vi "Write cRIO.vi"(10 "cRIO":T1={"Username"="admin", "IP Address"="140.252.33.38", "Path to ts_opensplice target"=path "/usr", "Path to ts_sal target"=path "/usr"}, 11 "FileTransfer in":refnum<class "FileTransfer.lvclass">) -> (3 "FileTransfer out":refnum<class "FileTransfer.lvclass">)   [LabVIEW 2016, in "FileTransfer.lvclass"]
uses:
  FileTransfer.lvclass
  Typedefs/cRIO.ctl
  FileTransfer.lvclass/FileTransfer.ctl
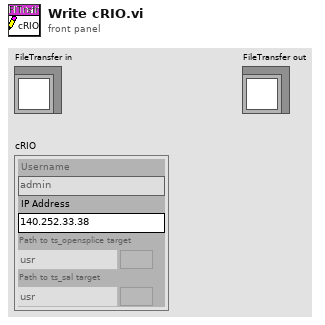
[diagram p1: front panel]
types:
  T1 = typedef "cRIO.ctl" = cluster{"Username":string, "IP Address":string, "Path to ts_opensplice target":path, "Path to ts_sal target":path}
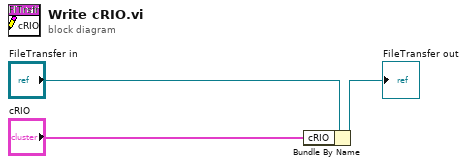
[diagram p0: block diagram]
diagram:
  n1 = Bundle By Name(cluster="FileTransfer in", "cRIO"="cRIO") -> (→"FileTransfer out":refnum<class "FileTransfer.lvclass">)
